vi "Dialog box to select a device_libESP301.vi"(6 "Error IN":errorcluster, 8 "Connected devices":string[](array[string]), 9 "Title":string) -> (0 "Error OUT":errorcluster, 1 "Controller address":i32=1, 2 "Selected device":string, 4 "OK?":bool)   [LabVIEW 2020, in "Newport ESP301.lvlib"]
doc: "Dialog box to select a CONEX device from a list."
uses:
  Newport ESP301.lvlib
panel:
  in  "Cancel":bool
  in  "Controller address":i32=1
  in  "Bouton OK":bool
  in  "COM Ports":i32(listbox)=-1 caption="Connected devices"
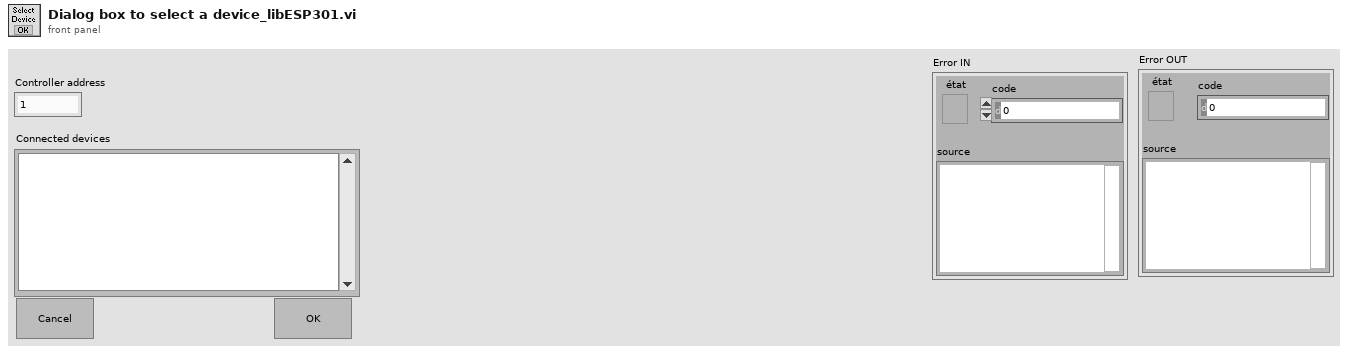
[diagram p1: front panel]
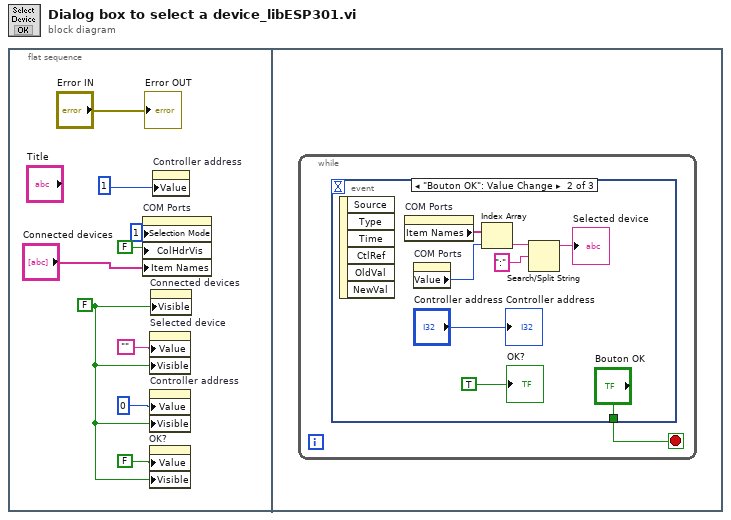
[diagram p0: block diagram]
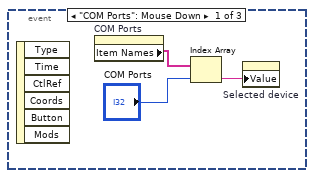
[diagram p2: hidden frame]
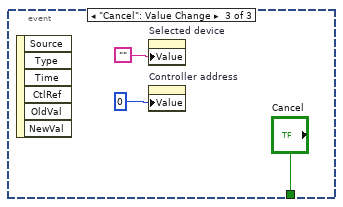
[diagram p3: hidden frame]
diagram:
  n1 = flat-sequence {
    frame #0 {
      w2 = FALSE ("Visible")
      n2 = property on="COM Ports" class="LstBox (strict)"("Selection Mode"=1, "ColHdrVis"=FALSE ("Éléments visibles : en-tête de colonne visible"), "Item Names"="Connected devices") -> ()  [unwired: 2 in, 2 out]
      n3 = property on="Selected device" class="Str"("Value"="", "Visible"=w2) -> ()  [unwired: 2 in, 2 out]
      n4 = property on="Controller address" class="DigNum (strict)"("Value"=0 ("Controller address"), "Visible"=w2) -> ()  [unwired: 2 in, 2 out]
      n5 = property on="OK?" class="Bool (strict)"("Value"=FALSE ("OK?"), "Visible"=w2) -> ()  [unwired: 2 in, 2 out]
      n6 = property on="Connected devices" class="Arr (strict)"("Visible"=w2) -> ()  [unwired: 2 in, 2 out]
      n7 = property on="Controller address" class="DigNum (strict)"("Value"=1 ("Controller address")) -> ()  [unwired: 2 in, 2 out]
      "Error OUT" <- "Error IN"
    }
    frame #1 {
      n8 = while {
        stop <- w10 stop-if-true
        n9 = event shown="[1] \"Bouton OK\": Value Change" {
          selector: _ -> [_ _ _]
          dyn-events: _ -> [_ _ _]
          timeout: _ -> [_ _ _]
          tunnel: [_ "Bouton OK" "Cancel"] -> w10
          event "COM Ports": Mouse Down {
            n10 = event-data() -> ()  [unwired: 7 out]
            n11 = property on="COM Ports" class="LstBox (strict)"() -> ("Item Names"=w12:string[])  [unwired: 2 in, 2 out]
            n12 = Index Array(array=w12, index="COM Ports") -> (element=w11:string)
            n13 = property on="Selected device" class="Str"("Value"=w11) -> ()  [unwired: 2 in, 2 out]
          }
          event "Bouton OK": Value Change {
            n14 = event-data() -> ()  [unwired: 7 out]
            n15 = property on="COM Ports" class="LstBox (strict)"() -> ("Item Names"=w16:string[])  [unwired: 2 in, 2 out]
            n16 = property on="COM Ports" class="LstBox (strict)"() -> ("Value"=w17:i32)  [unwired: 2 in, 2 out]
            n17 = Index Array(array=w16, index=w17) -> (element=w18:string)
            n18 = Search/Split String(string=w18, search string/char (-)=":" ("chaîne/car. recherché (-)")) -> (substring before match=→"Selected device":string)  [unwired: 3 out]
            "Controller address" <- "Controller address"
            "OK?" <- TRUE ("OK?")
          }
          event "Cancel": Value Change {
            n19 = event-data() -> ()  [unwired: 7 out]
            n20 = property on="Selected device" class="Str"("Value"="") -> ()  [unwired: 2 in, 2 out]
            n21 = property on="Controller address" class="DigNum (strict)"("Value"=0 ("Controller address")) -> ()  [unwired: 2 in, 2 out]
          }
        }
      }
    }
  }
